vi "总磷总氮公式写入.vi"(7 "公式":cluster{"X^2":dbl, "X":dbl, "b":dbl}, 8 "error in (no error)":errorcluster caption="错误输入（无错误）", 9 "量程":enum16{"低量程", "高量程"}(ring), 10 "测量模式":enum16{"水样测量", "零点核查", "跨度核查", "标样核查", "加标回收"}(ring), 11 "测量参数":enum16{"总磷", "总氮"}(ring)) -> (0 "error out":errorcluster caption="错误输出")   [LabVIEW 2016, in "斯坦道总氮.lvlib"]
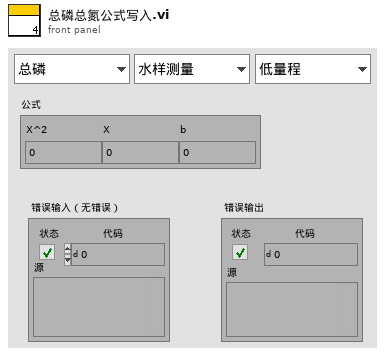
[diagram p1: front panel]
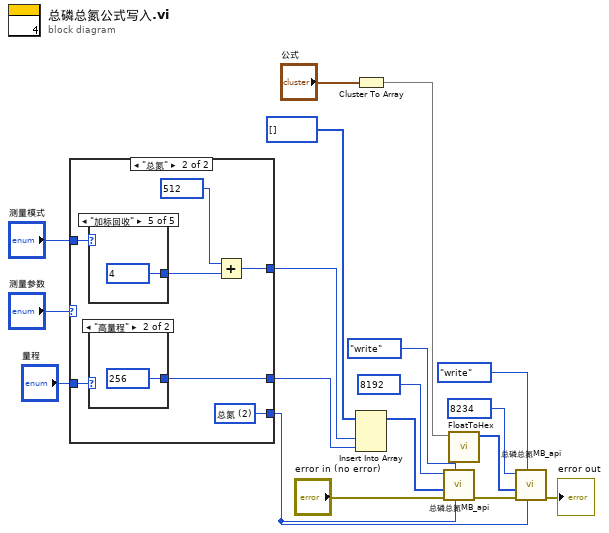
[diagram p0: block diagram]
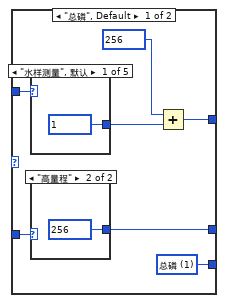
[diagram p2: hidden frame]
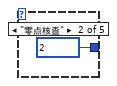
[diagram p3: hidden frame]
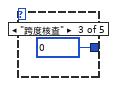
[diagram p4: hidden frame]
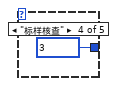
[diagram p5: hidden frame]
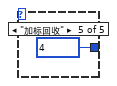
[diagram p6: hidden frame]
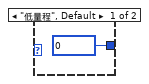
[diagram p7: hidden frame]
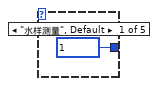
[diagram p8: hidden frame]
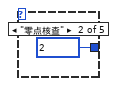
[diagram p9: hidden frame]
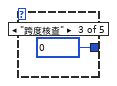
[diagram p10: hidden frame]
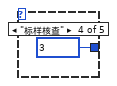
[diagram p11: hidden frame]
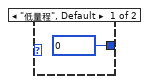
[diagram p12: hidden frame]
diagram:
  n1 = case shown="\"总氮\"" "测量参数" {
    tunnel: "测量模式" -> [w24 w37]
    tunnel: "量程" -> [w25 w38]
    tunnel: [w19 w39] -> w6
    tunnel: [w20 w33] -> w10
    tunnel: [w23 w36] -> w9
    frame "总磷", Default {
      w19 = u16 1 items=["总磷"=1, "总氮"=2, "氨氮"=3] ("站号")
      n2 = case shown="\"水样测量\", 默认" w24 {
        tunnel: [u16 1 ("starting address") u16 2 ("starting address") u16 0 ("starting address") u16 3 ("starting address") u16 4 ("starting address")] -> w22
        frame "水样测量", Default {
        }
        frame "零点核查" {
        }
        frame "跨度核查" {
        }
        frame "标样核查" {
        }
        frame "加标回收" {
        }
      }
      n3 = case shown="\"高量程\"" w25 {
        tunnel: [u16 0 ("starting address") u16 256 ("starting address")] -> w23
        frame "低量程", Default {
        }
        frame "高量程" {
        }
      }
      n4 = Add(x=u16 256 ("starting address"), y=w22) -> (x+y=w20:u16)
    }
    frame "总氮" {
      w39 = u16 2 items=["总磷"=1, "总氮"=2, "氨氮"=3] ("站号")
      n5 = case shown="\"加标回收\"" w37 {
        tunnel: [u16 1 ("starting address") u16 2 ("starting address") u16 0 ("starting address") u16 3 ("starting address") u16 4 ("starting address")] -> w35
        frame "水样测量", Default {
        }
        frame "零点核查" {
        }
        frame "跨度核查" {
        }
        frame "标样核查" {
        }
        frame "加标回收" {
        }
      }
      n6 = case shown="\"高量程\"" w38 {
        tunnel: [u16 0 ("starting address") u16 256 ("starting address")] -> w36
        frame "低量程", Default {
        }
        frame "高量程" {
        }
      }
      n7 = Add(x=u16 512 ("starting address"), y=w35) -> (x+y=w33:u16)
    }
  }
  n8 = Cluster To Array(cluster="公式") -> (array=w17:dbl[])
  n9 = Insert Into Array(array=u16[] [] ("数组"), new element #1=w10, new element #2=w9) -> (w2:u16[])  [unwired: 1 in]
  n10 = call "总磷总氮MB_api.vi"("Slave ID"=w6, "STEP"=enum16{"open", "read", "write", "close"}."write", "Error in"="error in (no error)", "values"=w2, "starting address"=u16 8192) -> ("error out"=w5:errorcluster)  [unwired: 4 in, 2 out]
  n11 = call "FloatToHex.vi"("浮点数"=w17) -> ("DCBA整形输出"=w1:u16[])  [unwired: 10 in]
  n12 = call "总磷总氮MB_api.vi"("Slave ID"=w6, "STEP"=enum16{"open", "read", "write", "close"}."write", "Error in"=w5, "values"=w1, "starting address"=u16 8234) -> ("error out"=→"error out":errorcluster)  [unwired: 4 in, 2 out]
